vi "Logging.Stop.vi"(8 "error in (no error)":errorcluster) -> (0 "error out":errorcluster)   [LabVIEW 2018]
uses:
  <vilib>/Field R&D Services/Logger/Private/Control State.vi
  <vilib>/Field R&D Services/Logger/Logger.lvlib
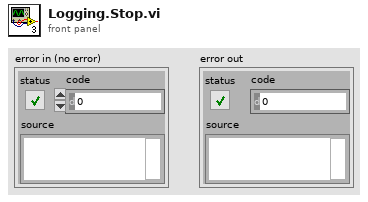
[diagram p1: front panel]
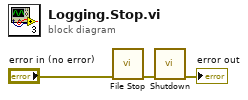
[diagram p0: block diagram]
diagram:
  n1 = call <vilib>:"File Stop.vi"("Error In"="error in (no error)") -> ("Error Out"=w3:errorcluster)  [unwired: 10 in]
  n2 = call <vilib>:"Shutdown.vi"("Error In"=w3) -> ("Error Out"=→"error out":errorcluster)  [unwired: 10 in]
